vi "Write Port Ref.vi"(8 "error in (no error)":errorcluster, 10 "Port Ref":refnum<visa-resource-name>, 11 "RS232 to GPIB ConvBox in":refnum<class "RSxxx to GPIB ConvBox.lvclass">) -> (0 "error out":errorcluster, 3 "RS232 to GPIB ConvBox out":refnum<class "RSxxx to GPIB ConvBox.lvclass">)   [LabVIEW 2019, in "Protocols.lvlib" / "RSxxx to GPIB ConvBox.lvclass"]
uses:
  RSxxx to GPIB ConvBox.lvclass
  RSxxx to GPIB ConvBox.lvclass/RSxxx to GPIB ConvBox.ctl
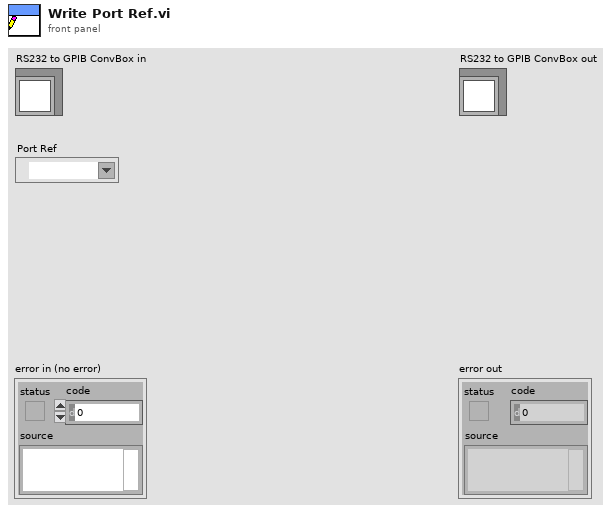
[diagram p1: front panel]
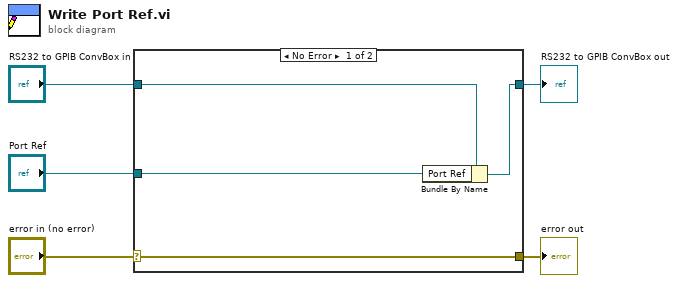
[diagram p0: block diagram]
diagram:
  n1 = case shown="No Error" "error in (no error)" {
    selector: "error in (no error)" -> [w9 w10]
    tunnel: [w9 w10] -> w4
    tunnel: [w7 w11] -> w2
    tunnel: "RS232 to GPIB ConvBox in" -> [w8 w11]
    tunnel: "Port Ref" -> [w6 _]
    frame No Error {
      n2 = Bundle By Name(cluster=w8, "Port Ref"=w6) -> (w7:refnum<class "RSxxx to GPIB ConvBox.lvclass">)
    }
    frame Error {
    }
  }
  "error out" <- w4
  "RS232 to GPIB ConvBox out" <- w2
